vi "Do.vi"(8 "error in (no error)":errorcluster, 10 "Actor in":refnum<class "Actor.lvclass">, 11 "Update Status Display":refnum<class "Update Status Display.lvclass">) -> (0 "error out":errorcluster, 2 "Actor out":refnum<class "Actor.lvclass">)   [LabVIEW 2016, in "Generic UI Actor.lvlib" / "Update Status Display.lvclass"]
uses:
  Update Status Display.lvclass
  <vilib>/ActorFramework/Actor/Actor.lvclass
  UI.lvclass
  C:/Program Files (x86)/National Instruments/LabVIEW 2016/vi.lib/ActorFramework/Actor/Actor.lvclass
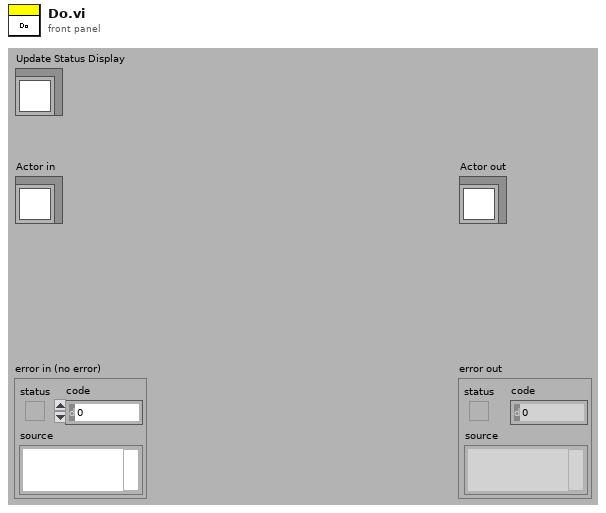
[diagram p1: front panel]
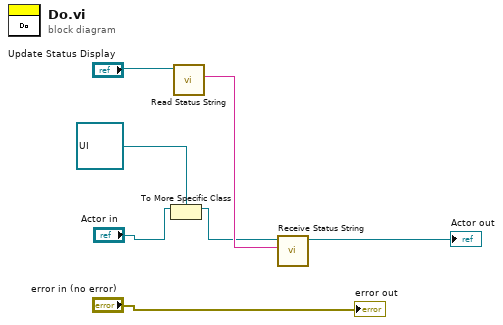
[diagram p0: block diagram]
diagram:
  n1 = To More Specific Class(target class=refnum<class "UI.lvclass"> refnum ("UI.lvclass"), reference="Actor in") -> (specific class reference=w2:refnum<class "UI.lvclass">)  [unwired: 1 in, 1 out]
  n2 = call "Read Status String.vi"("Update Status Display in"="Update Status Display") -> ("Status String"=w3:string)  [unwired: 8 in, 2 out]
  n3 = call-dynamic "Receive Status String.vi"("Status String"=w3, "UI in"=w2) -> ("UI out"=→"Actor out":refnum<class "UI.lvclass">)  [unwired: 8 in, 1 out]
  "error out" <- "error in (no error)"
